vi "VolumeFlowCalculator_2.vi"() -> ()   [LabVIEW 2013]
panel:
  out "Pressure 2":dbl
  out "Pressure 1":dbl
  out "Measured Voltage 2":dbl
  out "Measured Voltage":dbl
  out "?":dbl(slide) scale=0.0..40000.0
  out "?":dbl(slide) scale=0.0..10000.0
  out "?":dbl
  out "?":dbl
  out "?":dbl
  out "?":dbl
  in  "?":dbl(slide) scale=0.0..1000.0
  in  "Gas Constant":dbl(slide) scale=0.0..400.0
  in  "Coefficient of Outflow C":dbl(slide) scale=0.0..2.0
  in  "Density of Liquid":dbl(slide) scale=0.0..2.0
  in  "Diameter of Tube in Position 2":dbl(slide) scale=0.0..300.0
  in  "Diameter of Tube in Position 1":dbl(slide) scale=0.0..300.0
  in  "Gas/Liquid":bool
  # "ECE 4342: Lab 6 - Volumetric Flow Calculator - Spring 2015 - Abhishek Barla (ID: 900559822)"
  # "Inputs"
  # "Outputs"
  # "Velocity in Position 1"
  # "Velocity in Position 2"
  # "Liquid"
  # "mm"
  # "Gas"
  # "m/s"
  # "m/s"
  # "Volumetric Flow"
  # "l/s"
  # "Mass Flow"
  # "g/s"
  # "mm"
  # "Pa"
  # "V"
  # "Temperature"
  # "Pa"
  # "V"
  # "K"
  # "Kg/m^3"
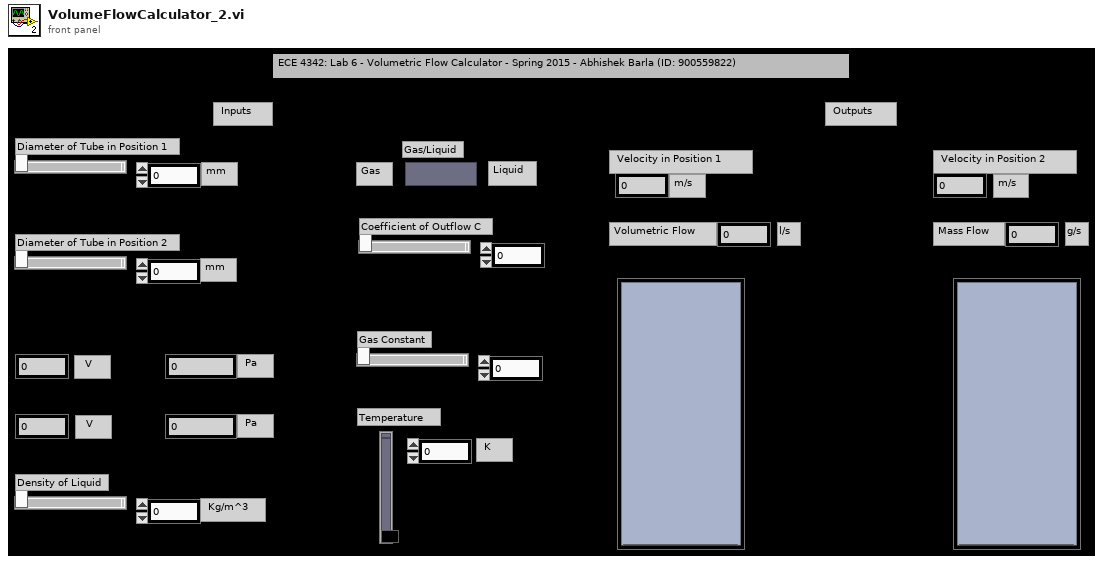
[diagram p1: front panel]
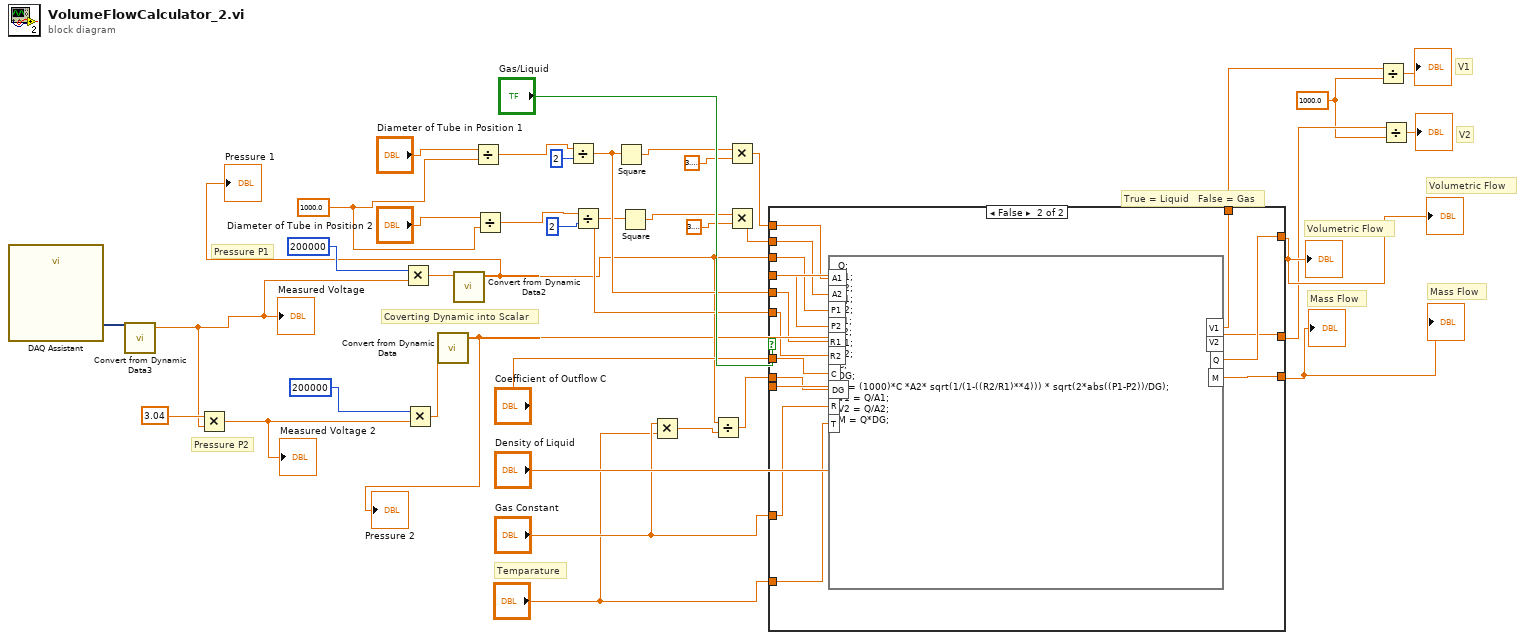
[diagram p0: block diagram]
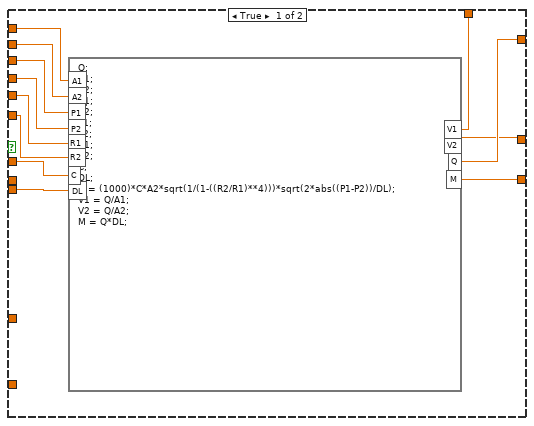
[diagram p2: hidden frame]
diagram:
  w11 = 1000.0
  w24 = 1000.0
  # "Coverting Dynamic into Scalar"
  # "Pressure P2"
  # "Pressure P1"
  # "Mass Flow"
  # "Volumetric Flow"
  # "True = Liquid   False = Gas"
  # "Volumetric Flow"
  # "V1"
  # "Mass Flow"
  # "V2"
  # "Temparature"
  n1 = call "DAQ Assistant"() -> ("data"=w6:dynamicdata)  [unwired: 17 in, 2 out]
  n2 = call "Convert from Dynamic Data3"("Dynamic Data Type"=w6) -> ("Scalar"=w4:dbl)  [unwired: 3 in]
  "Measured Voltage" <- w4
  n3 = Multiply(x=3.04, y=w4) -> (x*y=w3:dbl)
  "Measured Voltage 2" <- w3
  n4 = Multiply(x=200000, y=w4) -> (x*y=w7:dbl)
  n5 = Multiply(x=200000, y=w3) -> (x*y=w8:dbl)
  n6 = call "Convert from Dynamic Data"("Dynamic Data Type"=w8) -> ("Scalar"=w1:dbl)  [unwired: 3 in]
  "Pressure 2" <- w1
  n7 = call "Convert from Dynamic Data2"("Dynamic Data Type"=w7) -> ("Scalar"=w2:dbl)  [unwired: 3 in]
  "Pressure 1" <- w2
  n8 = Divide(x="Diameter of Tube in Position 1", y=w24) -> (x/y=w22:dbl)
  n9 = Divide(x="Diameter of Tube in Position 2", y=w24) -> (x/y=w23:dbl)
  n10 = Divide(x=w22, y=2) -> (x/y=w31:dbl)
  n11 = Divide(x=w23, y=2) -> (x/y=w30:dbl)
  n12 = Square(x=w31) -> (x^2=w36:dbl)
  n13 = Square(x=w30) -> (x^2=w35:dbl)
  n14 = Multiply(x="Gas Constant", y="?") -> (x*y=w17:dbl)
  n15 = Divide(x=w2, y=w17) -> (x/y=w16:dbl)
  n16 = Multiply(x=w36, y=3.141592653589793) -> (x*y=w33:dbl)
  n17 = Multiply(x=w35, y=3.141592653589793) -> (x*y=w32:dbl)
  n18 = case shown="False" "Gas/Liquid" {
    tunnel: w33 -> [w51 w65]
    tunnel: w32 -> [w50 w64]
    tunnel: w2 -> [w49 w63]
    tunnel: w1 -> [w48 w62]
    tunnel: w31 -> [w47 w61]
    tunnel: w30 -> [w46 w60]
    tunnel: [w45 w59] -> w28
    tunnel: "Density of Liquid" -> [w44 _]
    tunnel: "Coefficient of Outflow C" -> [w43 w58]
    tunnel: [w42 w57] -> w15
    tunnel: [w41 w56] -> w14
    tunnel: [w40 w55] -> w27
    tunnel: "Gas Constant" -> [_ w54]
    tunnel: "?" -> [_ w53]
    tunnel: w16 -> [_ w52]
    frame True {
      n19 = formula code="Q;\nA1;\nA2;\nV1;\nV2;\nP1;\nP2;\nR1;\nR2;\nC;\nDL;\nQ = (1000)*C*A2*sqrt(1/(1-((R2/R1)**4)))*sqrt(2*abs((P1-P2))/DL);\nV1 = Q/A1;\nV2 = Q/A2;\nM = Q*DL;"("A1"=w51, "A2"=w50, "P1"=w49, "P2"=w48, "R1"=w47, "R2"=w46, "DL"=w44, "C"=w43) -> ("Q"=w45:dbl, "V2"=w41:dbl, "V1"=w42:dbl, "M"=w40:dbl)
    }
    frame False {
      n20 = formula code="Q;\nA1;\nA2;\nV1;\nV2;\nP1;\nP2;\nR1;\nR2;\nC;\nDG; \nQ = (1000)*C *A2* sqrt(1/(1-((R2/R1)**4))) * sqrt(2*abs((P1-P2))/DG);\nV1 = Q/A1;\nV2 = Q/A2;\nM = Q*DG;"("A1"=w65, "A2"=w64, "P1"=w63, "P2"=w62, "R1"=w61, "R2"=w60, "C"=w58, "R"=w54, "T"=w53, "DG"=w52) -> ("Q"=w59:dbl, "V2"=w56:dbl, "V1"=w57:dbl, "M"=w55:dbl)
    }
  }
  "?" <- w28
  "?" <- w27
  "?" <- w28
  "?" <- w27
  n21 = Divide(x=w15, y=w11) -> (x/y=→"?":dbl)
  n22 = Divide(x=w14, y=w11) -> (x/y=→"?":dbl)
